vi "Initialize MeasurementLink Session.vi"(7 "remote connection options":T2, 8 "error in":errorcluster, 9 "initialize and close session behavior":T1, 10 "session initialization parameters":T3, 11 "session factory in":refnum<class "Session Factory.lvclass">) -> (0 "error out":errorcluster, 2 "session out":variant, 3 "session factory out":refnum<class "Session Factory.lvclass">)   [LabVIEW 2020, in "niDMM Sessions.lvlib" / "Session Factory.lvclass"]
uses:
  Session Factory.lvclass
  Instrument Sessions/ISession Factory/Session Initialization Parameters.ctl
  Instrument Sessions/ISession Factory/Remote Connection Options.ctl
  Instrument Sessions/ISession Factory/Initialize and Close Session Behavior.ctl
  Session Factory.lvclass/Session Factory.ctl
  Instrument Sessions/ISession Factory/ISession Factory.lvclass
  <instrlib>/niDMM/nidmm.llb/niDMM Initialize for gRPC Session.vi
  <instrlib>/niDMM/nidmm.llb/niDMM Attach gRPC Session.vi
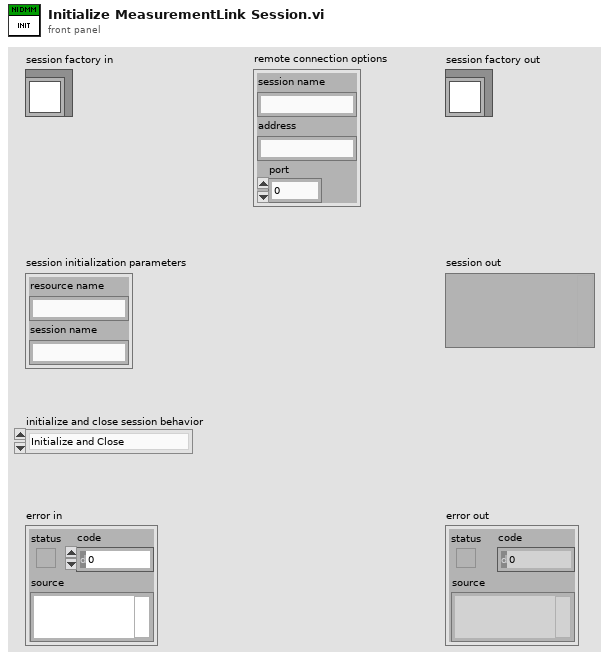
[diagram p1: front panel]
types:
  T1 = typedef "Instrument Sessions.lvlib/ISession Factory.lvclass/Initialize and Close Session Behavior.ctl" = enum16{"Initialize and Close", "Attach and Detach", "Initialize and Detach", "Attach and Close"}
  T2 = typedef "Instrument Sessions.lvlib/ISession Factory.lvclass/Remote Connection Options.ctl" = cluster{"session name":string, "address":string, "port":u32}
  T3 = typedef "Instrument Sessions.lvlib/ISession Factory.lvclass/Session Initialization Parameters.ctl" = cluster{"resource name":string, "session name":string}
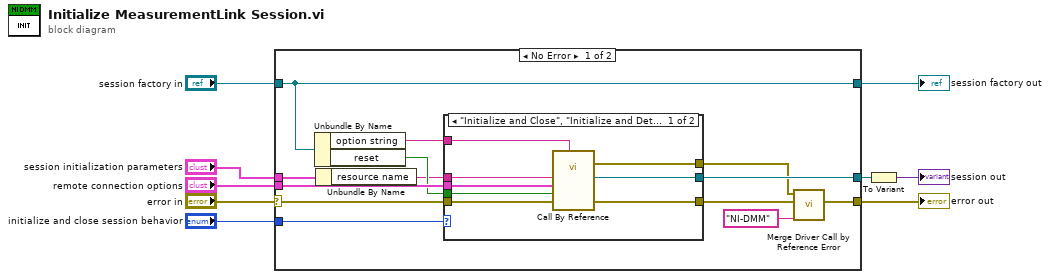
[diagram p0: block diagram]
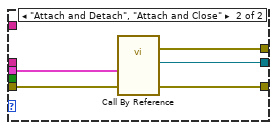
[diagram p2: hidden frame]
diagram:
  n1 = case shown="No Error" "error in" {
    selector: "error in" -> [w19 w36]
    tunnel: [w11 w36] -> w8
    tunnel: "session factory in" -> [w17 w37]
    tunnel: [w17 w37] -> w6
    tunnel: "initialize and close session behavior" -> [w22 _]
    tunnel: "remote connection options" -> [w21 _]
    tunnel: "session initialization parameters" -> [w18 _]
    tunnel: [w20 _] -> w2
    frame No Error {
      n2 = Unbundle By Name(w17) -> ("option string"=w16:string, "reset"=w15:bool)
      n3 = Unbundle By Name(w18) -> ("resource name"=w14:string)
      n4 = case shown="\"Initialize and Close\", \"Initialize and Detach\"" w22 {
        tunnel: w21 -> [w29 w35]
        tunnel: [w28 w34] -> w20
        tunnel: w19 -> [w30 w33]
        tunnel: [w27 w32] -> w12
        tunnel: w14 -> [w26 _]
        tunnel: w16 -> [w25 _]
        tunnel: w15 -> [w24 _]
        tunnel: [w23 w31] -> w10
        frame "Initialize and Close", "Initialize and Detach" {
          n5 = call-by-ref "?"("Option String"=w25, "error in (no error)"=w30, "Reset Device"=w24, "gRPC Options"=w29, "Instrument Descriptor"=w26) -> (error out=w23:errorcluster, 0:"error out"=w27:errorcluster, "instrument handle out"=w28:refnum<k15>)  [unwired: 7 in, 1 out]
        }
        frame "Attach and Detach", "Attach and Close" {
          n6 = call-by-ref "?"("error in (no error)"=w33, "gRPC Options"=w35) -> (error out=w31:errorcluster, 0:"error out"=w32:errorcluster, "instrument handle out"=w34:refnum<k15>)  [unwired: 10 in, 1 out]
        }
      }
      n7 = call "Merge Driver Call by Reference Error.vi"("driver name"="NI-DMM", "called vi error"=w12, "call by ref error"=w10) -> ("error out"=w11:errorcluster)  [unwired: 8 in]
    }
    frame Error {
    }
  }
  "error out" <- w8
  "session factory out" <- w6
  n8 = To Variant(anything=w2) -> (Variant=→"session out":variant)
